vi "Write Running Methods Communication.vi"(8 "error in (no error)":errorcluster, 10 "Running Methods Communication":T1, 11 "Async Methods Actor in":refnum<class "Async Methods Actor.lvclass">) -> (0 "error out":errorcluster, 3 "Async Methods Actor out":refnum<class "Async Methods Actor.lvclass">)   [LabVIEW 2023, in "Async Methods Actor.lvlib" / "Async Methods Actor.lvclass"]
doc: "This property allows setting up a communication method based either on a notifier or an event structure that allows the subscriber to receive information about the Async Messages currently running. The subscriber will receive the FQN of the running Async Messages, the number of running Async Messages launched by the \"Call & Collect\" method and the number of launched Async Messages launched by the \"Call & Collect\" method. The setting is controlled by the \"\" enum that can take values \"None\" (default), \"Notifier\" and \"Event\": the first disables the communication, the second sets it up by means of a notifier that can be accessed by means of the \"Async Messages Running Notifier\" while the third sets it up by means of a event mechanism whose reference can be accessed by means of the \"Async Messages Running Event Ref\"."
uses:
  Async Methods Actor.lvclass
  Running Methods Communication.ctl
  Async Methods Actor.lvclass/Async Methods Actor.ctl
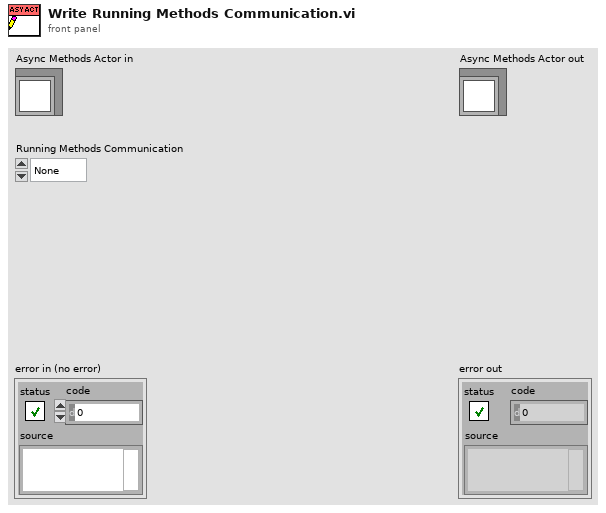
[diagram p1: front panel]
types:
  T1 = typedef "Async Methods Actor.lvlib/Async Methods Actor.lvclass/Running Methods Communication.ctl" = enum16{"None", "Notifier", "Event"}
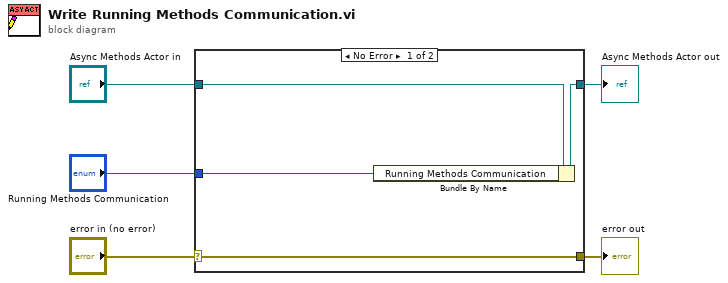
[diagram p0: block diagram]
diagram:
  n1 = case shown="No Error" "error in (no error)" {
    selector: "error in (no error)" -> [w9 w10]
    tunnel: [w9 w10] -> w4
    tunnel: [w7 w11] -> w2
    tunnel: "Async Methods Actor in" -> [w8 w11]
    tunnel: "Running Methods Communication" -> [w6 _]
    frame No Error {
      n2 = Bundle By Name(cluster=w8, "Running Methods Communication"=w6) -> (w7:refnum<class "Async Methods Actor.lvclass">)
    }
    frame Error {
    }
  }
  "error out" <- w4
  "Async Methods Actor out" <- w2
